vi "path reader.vi"(2 "Iterations":i32, 3 "Path":path) -> (0 "Angular Data":dbl[](array[numeric]), 1 "Velocity Data":dbl[](array[numeric]))   [LabVIEW 2018]
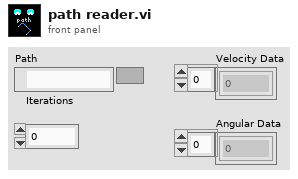
[diagram p1: front panel]
types:
  T1 = cluster{"Segment Name":string, "Type":enum16{"Accel Straight", "Const Straight", "Blend", "Circle"}, "Traj Pos Points":cluster{"x":dbl, "y":dbl, "th":dbl}[], "Traj Vel Points":cluster{"V":dbl, "th":dbl}[], "Accel Index":i32, "Decel Index":i32}[]
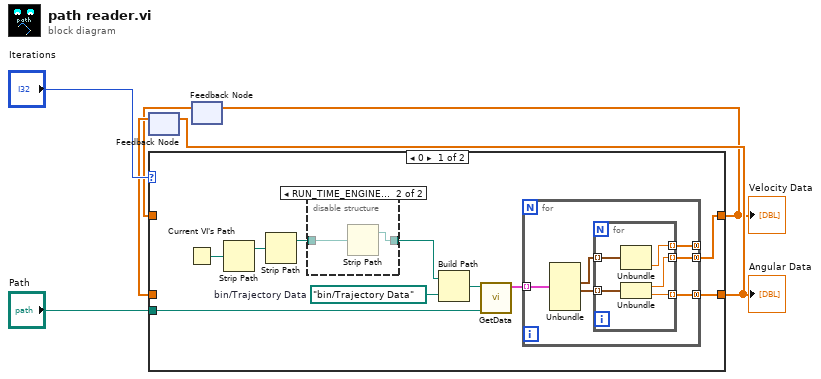
[diagram p0: block diagram]
diagram:
  n1 = feedback #1() -> (w2:dbl[])  [unwired: 1 in]
  n2 = feedback #2() -> (w1:dbl[])  [unwired: 1 in]
  n3 = case shown="0" "Iterations" {
    tunnel: [w16 w32] -> w3
    tunnel: [w15 w31] -> w6
    tunnel: w1 -> [_ w32]
    tunnel: w2 -> [_ w31]
    tunnel: "Path" -> [w9 _]
    frame 0 {
      w10 = path "bin/Trajectory Data"  # bin/Trajectory Data
      n4 = Current VI's Path() -> (path=w12:path)
      n5 = Strip Path(path=w12) -> (stripped path=w11:path)  [unwired: 1 out]
      n6 = Strip Path(path=w11) -> (stripped path=w7:path)  [unwired: 1 out]
      n7 = disable-structure shown="RUN_TIME_ENGINE==True, Default" {
        disable-tunnel: [w17 w18] -> w8
        disable-tunnel: w7 -> [w17 w19]
        frame condition #0 (active) {
        }
        frame condition #1 {
          n8 = Strip Path(path=w19) -> (stripped path=w18:path)  [unwired: 1 out]
        }
      }
      n9 = Build Path(base path=w8, name or relative path=w10) -> (appended path=w13:path)
      n10 = call "GetData.vi"("File"=w9, "file (use dialog)"=w13) -> ("Trajectory Data"=w14:T1)  [unwired: 3 in, 6 out]
      n11 = for {
        tunnel: [w25] -> w16 mode=concatenating
        tunnel: [w24] -> w15 mode=concatenating
        tunnel: w14 -> [w22] mode=indexing
        tunnel: [w21] -> _ mode=concatenating
        n12 = Unbundle(w22) -> ("Traj Pos Points"=w20:cluster{"x":dbl, "y":dbl, "th":dbl}[], "Traj Vel Points"=w23:cluster{"V":dbl, "th":dbl}[])  [unwired: 4 out]
        n13 = for {
          tunnel: w23 -> [w28] mode=indexing
          tunnel: [w30] -> w25 mode=indexing
          tunnel: [w29] -> w24 mode=indexing
          tunnel: w20 -> [w27] mode=indexing
          tunnel: [w26] -> w21 mode=indexing
          n14 = Unbundle(w27) -> ("th"=w26:dbl)  [unwired: 2 out]
          n15 = Unbundle(w28) -> ("V"=w30:dbl, "th"=w29:dbl)
        }
      }
    }
    frame 1, Default {
    }
  }
  "Angular Data" <- w6
  "Velocity Data" <- w3
  n16 = feedback-in #1(w6) -> ()
  n17 = feedback-in #2(w3) -> ()
